vi "DeleteDuplicateRefs.vi"(9 "CtrlRefs":refnum<vi>[](array[refnum]), 10 "DataType":T1[](array[typedef]), 11 "CtrlNames":string[](array[string])) -> (1 "CtrlRefs out":refnum<vi>[](array[refnum]), 2 "DataType out":T1[](array[typedef]), 3 "CtrlNames out":string[](array[string]))   [LabVIEW 2018, in "UI_Library.lvlib" / "UI_Library.lvclass"]
doc: "Remove duplicate from input array"
uses:
  UI_Library.lvclass
  <userlib>/_OpenG.lib/array/array.llb/openg_array.lvlib
  <userlib>/_OpenG.lib/array/array.llb/Remove Duplicates from 1D Array (String)__ogtk.vi
  <vilib>/Utility/Data Type/Type Definitions/Data Type.ctl
  <vilib>/Utility/Data Type/NI_Data Type.lvlib
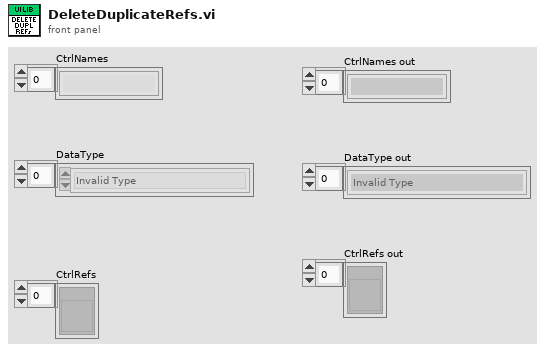
[diagram p1: front panel]
types:
  T1 = typedef "NI_Data Type.lvlib/Data Type.ctl" = enum8{"Invalid Type", "Void", "I8", "I16", "I32", "I64", "U8", "U16", "U32", "U64", "Single Float", "Double Float", "Extended Float", "Single Complex", "Double Complex", "Extended Complex", "Enum U8", "Enum U16", "Enum U32", "Enum U64", "Single Float With Unit", "Double Float With Unit", "Extended Float With Unit", "Single Complex with Unit", "Double Complex with Unit", "Extended Complex with Unit", "Boolean", "String", "Path", "Picture", "Tag", "Array", "Cluster", "Variant", "LV Variant", "Waveform", "Timestamp", "Digital Waveform", "Digital Data", "ExpressData", "Refnum", "External Data", "VI", "Poly VI", "LabVIEW Class Instance", "Fixed Point", "Set Collection", "Map Collection"}
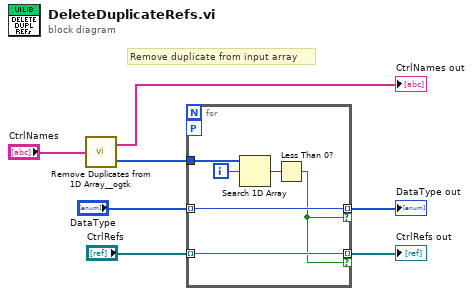
[diagram p0: block diagram]
diagram:
  # "Remove duplicate from input array"
  n1 = call-poly <userlib>:"Remove Duplicates from 1D Array__ogtk.vi"("Input Array"="CtrlNames") -> ("Output Array"=→"CtrlNames out":string[], "indices of removed elements"=w5:i32[])
  n2 = for {
    tunnel: w5 -> [w12]
    tunnel: "DataType" -> [w13] mode=indexing
    tunnel: [w13] -> w4 mode=indexing if=w8
    tunnel: "CtrlRefs" -> [w9] mode=indexing
    tunnel: [w9] -> w7 mode=indexing if=w8
    workers-P: _ -> [_]
    i -> [w11]
    n3 = Search 1D Array(1D array=w12, element=w11) -> (index of element=w10:i32)  [unwired: 1 in]
    n4 = Less Than 0?(x=w10) -> (x < 0?=w8:bool)
  }
  "CtrlRefs out" <- w7
  "DataType out" <- w4
